vi "OPC UA Server.vi"() -> ()   [LabVIEW 2017]
uses:
  <vilib>/OPCUA/controls/NodeId.ctl
  <vilib>/OPCUA/controls/Data Type.ctl
  <vilib>/OPCUA/NI OPC UA Server.lvlib
panel:
  out "item node ID":T1
  in  "stop":bool
  out "server endpoint URL":string
  out "error out":errorcluster
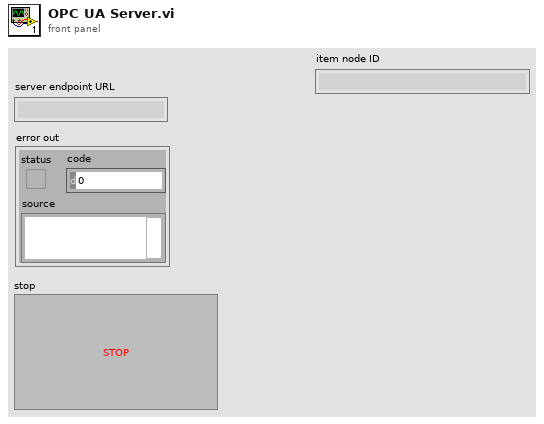
[diagram p1: front panel]
types:
  T1 = typedef "NodeId.ctl" = string
  T2 = typedef "Data Type.ctl" = u16
  T3 = cluster{"name":string, "data type":T2, "access level":u16, "description":string}
  T4 = typedef "OPC UA Server Refnum.ctl" = refnum<k21>
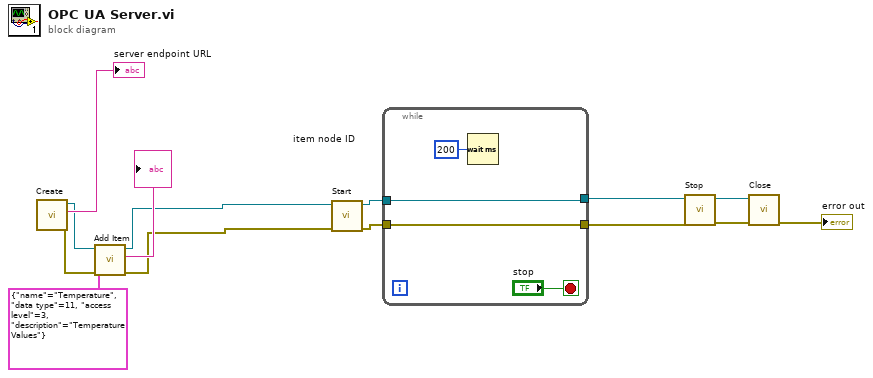
[diagram p0: block diagram]
diagram:
  n1 = call <vilib>:"Create.vi"() -> ("error out"=w7:errorcluster, "server endpoint URL"=→"server endpoint URL":string, "OPC UA server refnum out"=w8:T4)  [unwired: 9 in]
  n2 = call <vilib>:"Add Item.vi"("error in (no error)"=w7, "item"=T3 {"name"="Temperature", "data type"=11, "access level"=3, "description"="Temperature Values"}, "OPC UA server refnum in"=w8) -> ("error out"=w1:errorcluster, "item node ID"=→"item node ID":T1, "OPC UA server refnum out"=w2:T4)  [unwired: 4 in, 1 out]
  n3 = call <vilib>:"Start.vi"("error in (no error)"=w1, "OPC UA server refnum in"=w2) -> ("error out"=w3:errorcluster, "OPC UA server refnum out"=w4:T4)  [unwired: 7 in, 1 out]
  n4 = while {
    tunnel: [w18] -> w12
    tunnel: w4 -> [w18]
    tunnel: [w17] -> w11
    tunnel: w3 -> [w17]
    stop <- "stop" stop-if-true
    n5 = Wait (ms)(milliseconds to wait=u32 200) -> ()  [unwired: 1 out]
  }
  n6 = call <vilib>:"Stop.vi"("error in (no error)"=w11, "OPC UA server refnum in"=w12) -> ("error out"=w14:errorcluster, "OPC UA server refnum out"=w13:T4)  [unwired: 8 in]
  n7 = call <vilib>:"Close.vi"("error in (no error)"=w14, "OPC UA server refnum in"=w13) -> ("error out"=→"error out":errorcluster)  [unwired: 9 in]
